vi "InsertQuery.vi"(8 "Error In":errorcluster, 10 "input cluster":T1, 11 "connection reference":T2) -> (0 "Error Out":errorcluster, 2 "Result_2D":string[][](array[string]), 4 "Result_1D":string[](array[string]), 5 "Element":string, 6 "Result_1D Row":string[](array[string]))   [LabVIEW 2020]
uses:
  <vilib>/addons/database/Connection.llb/Conn ObjectReference.ctl
  crearQry.dll
  <vilib>/addons/database/Connection.llb/Conn Execute.vi
  <vilib>/addons/database/Recordset.llb/Rec Fetch Recordset Data (R).vi
  <vilib>/addons/database/Recordset.llb/Rec Destroy - Connection.vi
  <vilib>/addons/database/_DB Variant To Data/Database Variant To Data.xnode
  <vilib>/addons/database/NI_Database_API.lvlib
panel:
  out "Records":i32
  out "sqlQry":string
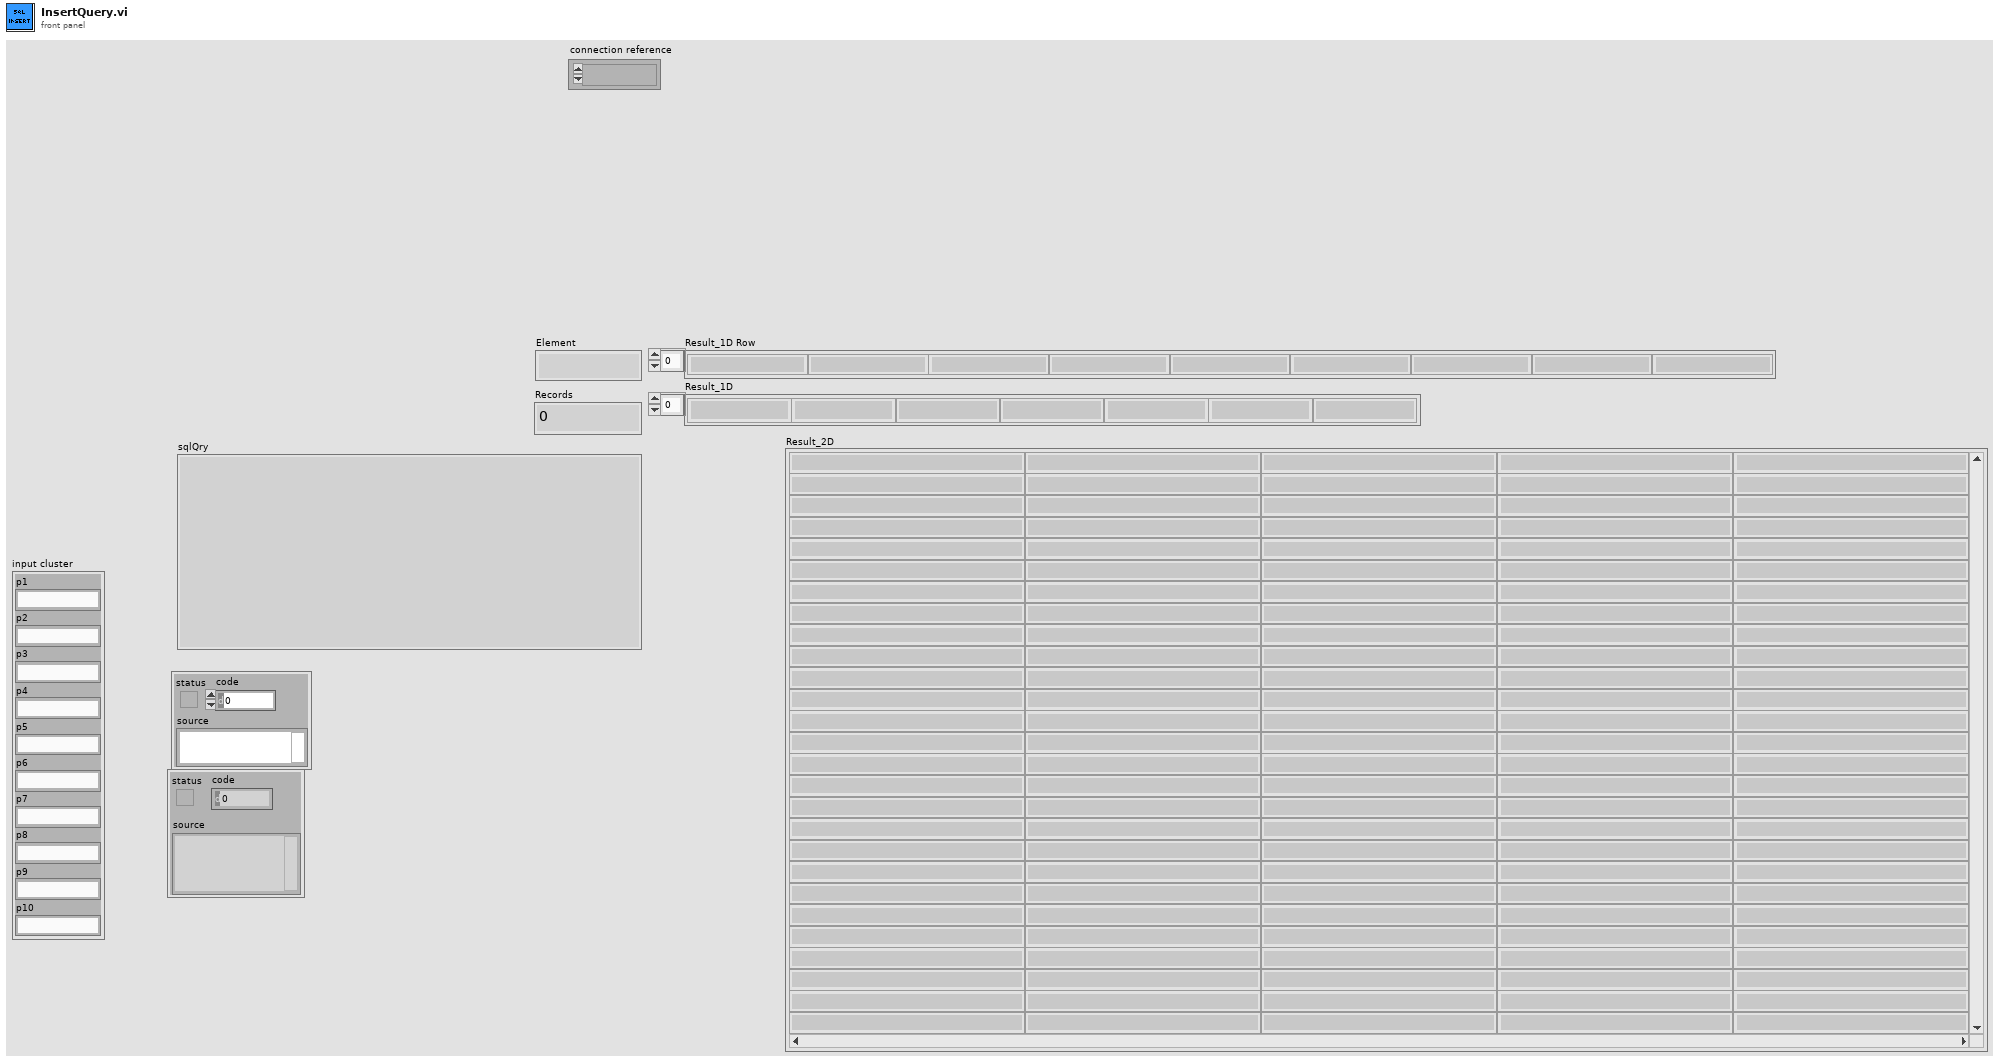
[diagram p1: front panel]
types:
  T1 = cluster{"p1":string, "p2":string, "p3":string, "p4":string, "p5":string, "p6":string, "p7":string, "p8":string, "p9":string, "p10":string}
  T2 = typedef "NI_Database_API.lvlib/Conn ObjectReference.ctl" = refnum<k1>
  T3 = typedef "NI_Database_API.lvlib/Rec ObjectReference.ctl" = refnum<k1>
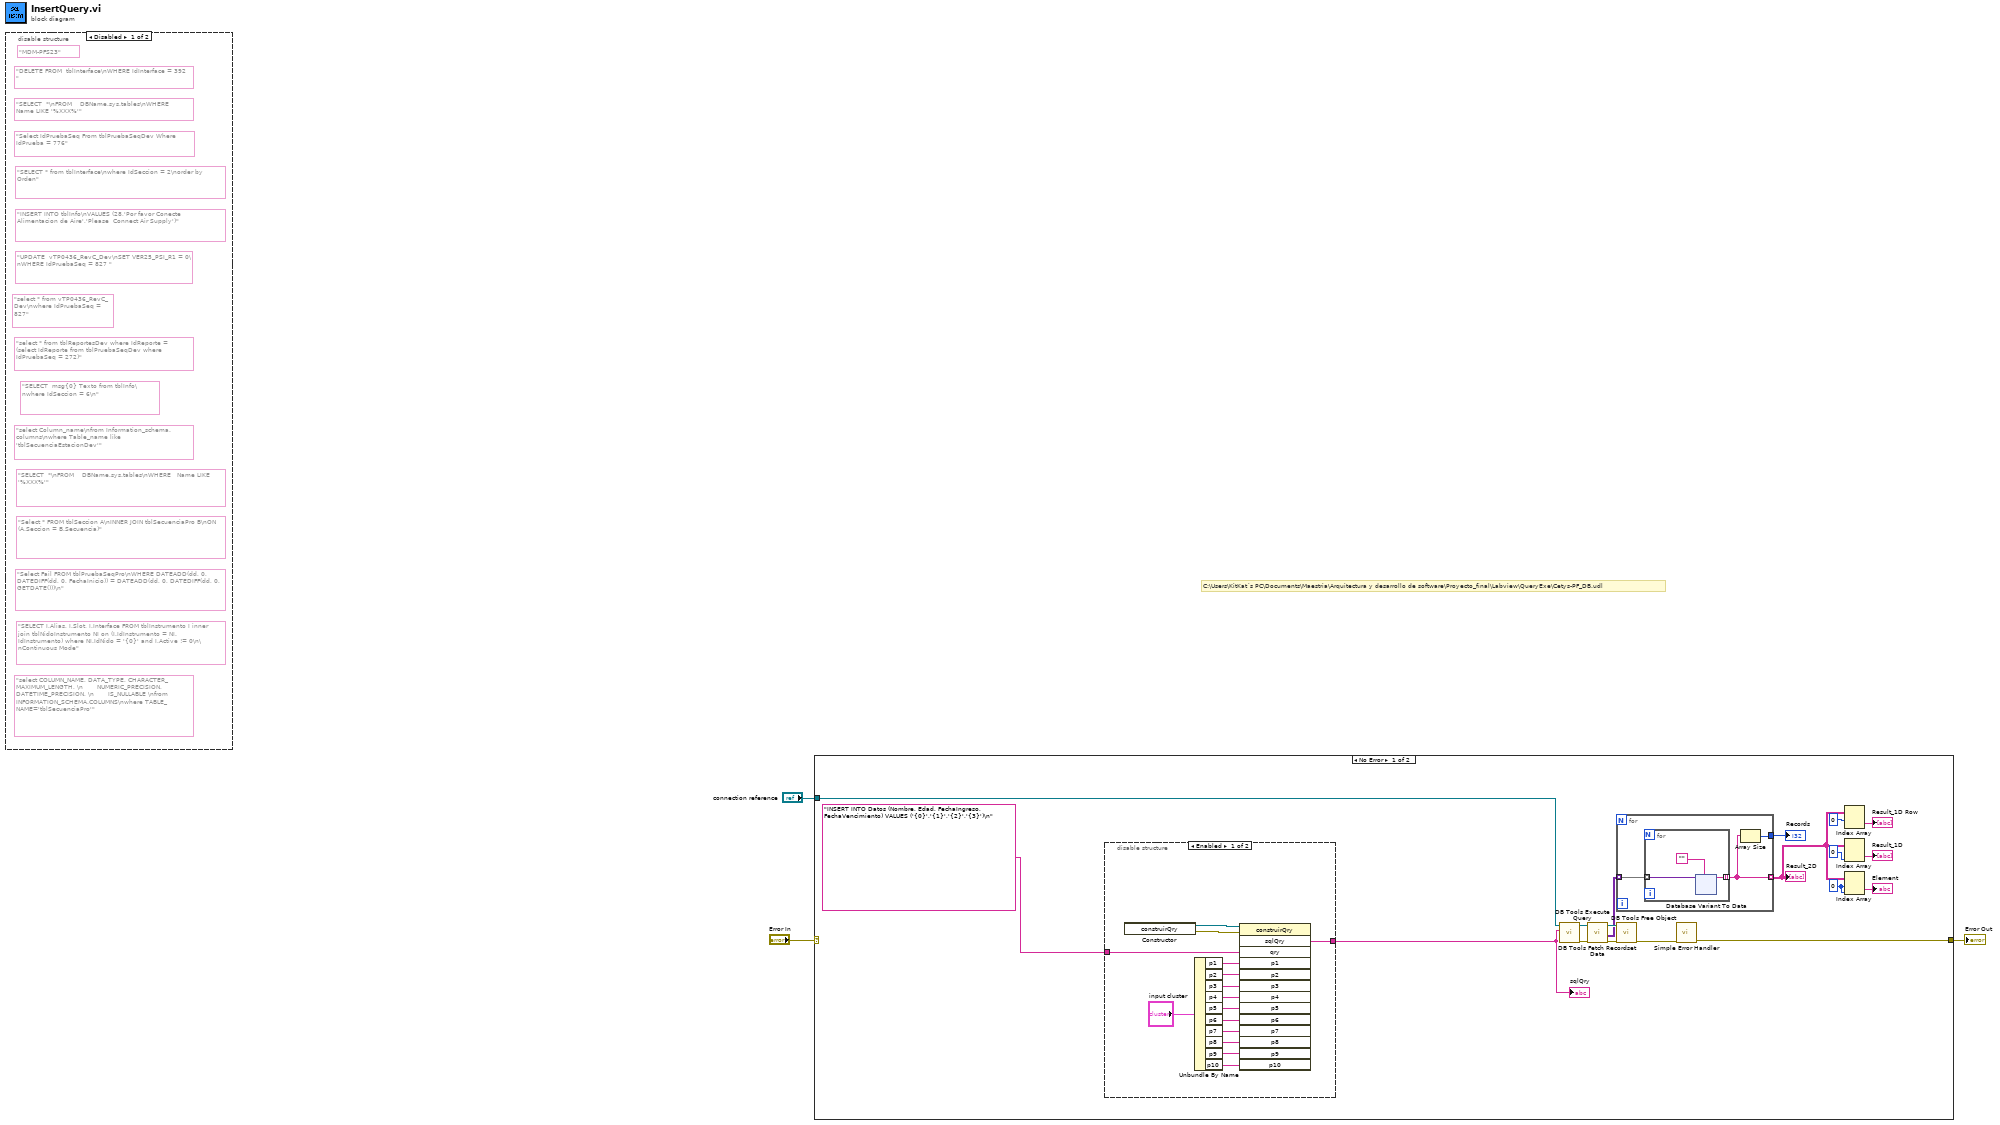
[diagram p0: block diagram]
diagram:
  # "C:\\Users\\KitKat´s PC\\Documents\\Maestria\\Arquitectura y desarrollo de software\\Proyecto_final\\Labview\\QueryExe\\Cetys-PF_DB.udl"
  n1 = disable-structure shown="Disabled" {
    frame Disabled {
      (unwired) "SELECT  msg{0} Texto from tblInfo\nwhere IdSeccion = 6\n" ("qry")
      (unwired) "select * from vTP0436_RevC_Dev\nwhere IdPruebaSeq = 827" ("qry")
      (unwired) "MDM-PFS23" ("Nombre de PC")
      (unwired) "SELECT  *\nFROM    DBName.sys.tables\nWHERE   Name LIKE '%XXX%'" ("qry")
      (unwired) "Select Fail FROM tblPruebaSeqPro\nWHERE DATEADD(dd, 0, DATEDIFF(dd, 0, FechaInicio)) = DATEADD(dd, 0, DATEDIFF(dd, 0, GETDATE()))\n" ("qry")
      (unwired) "Select * FROM tblSeccion A\nINNER JOIN tblSecuenciaPro B\nON (A.Seccion = B.Secuencia)" ("qry")
      (unwired) "SELECT * from tblInterface\nwhere IdSeccion = 2\norder by Orden" ("qry")
      (unwired) "SELECT I.Alias, I.Slot, I.Interface FROM tblInstrumento I inner join tblNidoInstrumento NI on (I.IdInstrumento = NI.IdInstrumento) where NI.IdNido = '{0}' and I.Active != 0\n\nContinuous Mode" ("qry")
      (unwired) "select * from tblReportesDev where IdReporte = (select IdReporte from tblPruebaSeqDev where IdPruebaSeq = 272)" ("sqlQry")
      (unwired) "DELETE FROM  tblInterface\nWHERE IdInterface = 392 " ("qry")
      (unwired) "select COLUMN_NAME, DATA_TYPE, CHARACTER_MAXIMUM_LENGTH, \n       NUMERIC_PRECISION, DATETIME_PRECISION, \n       IS_NULLABLE \nfrom INFORMATION_SCHEMA.COLUMNS\nwhere TABLE_NAME='tblSecuenciaPro'" ("qry")
      (unwired) "SELECT  *\nFROM    DBName.sys.tables\nWHERE   Name LIKE '%XXX%'" ("qry")
      (unwired) "select Column_name\nfrom Information_schema.columns\nwhere Table_name like 'tblSecuenciaEstacionDev'" ("qry")
      (unwired) "Select IdPruebaSeq From tblPruebaSeqDev Where IdPrueba = 776" ("qry")
      (unwired) "UPDATE  vTP0436_RevC_Dev\nSET VER25_PSI_R1 = 0\nWHERE IdPruebaSeq = 827 " ("qry")
      (unwired) "INSERT INTO tblInfo\nVALUES (28,'Por favor Conecte Alimentacion de Aire','Please  Connect Air Supply')" ("qry")
    }
    frame Enabled {
    }
  }
  n2 = case shown="No Error" "Error In" {
    selector: "Error In" -> [_ w75]
    tunnel: [w17 w75] -> w3
    tunnel: "connection reference" -> [w7 _]
    frame No Error {
      w14 = 0 ("index (row)")
      n3 = disable-structure shown="Enabled" {
        disable-tunnel: [w34 _] -> w5
        disable-tunnel: "INSERT INTO Datos (Nombre, Edad, FechaIngreso, FechaVencimiento) VALUES ('{0}','{1}','{2}','{3}')\n" ("qry") -> [w23 _]
        frame Enabled {
          n4 = constructor class="construirQry"() -> (reference out=w36:refnum<k24>, error out=w35:errorcluster)  [unwired: 3 in, 1 out]
          n5 = Unbundle By Name("input cluster") -> ("p1"=w33:string, "p2"=w32:string, "p3"=w31:string, "p4"=w30:string, "p5"=w29:string, "p6"=w28:string, "p7"=w27:string, "p8"=w26:string, "p9"=w25:string, "p10"=w24:string)
          n6 = invoke class="construirQry" method="sqlQry"(reference=w36, error in=w35, "qry"=w23, "p1"=w33, "p2"=w32, "p3"=w31, "p4"=w30, "p5"=w29, "p6"=w28, "p7"=w27, "p8"=w26, "p9"=w25, "p10"=w24) -> ("sqlQry"=w34:string)  [unwired: 1 in, 13 out]
        }
        frame Disabled {
        }
      }
      "sqlQry" <- w5
      n7 = call-poly <vilib>:"DB Tools Execute Query.vi"("SQL query"=w5, "connection reference"=w7) -> ("error out"=w20:errorcluster, "recordset reference"=w21:T3)  [unwired: 6 in]
      n8 = call-poly <vilib>:"DB Tools Fetch Recordset Data.vi"("error in (no error)"=w20, "recordset reference"=w21) -> ("error out"=w18:errorcluster, "recordset data"=w16:variant[][], "recordset reference out"=w19:T3)  [unwired: 3 in]
      n9 = for {
        tunnel: w16 -> [w39] mode=indexing
        tunnel: [w38] -> w10 mode=indexing
        tunnel: [w37] -> w15
        n10 = for {
          tunnel: w39 -> [w42] mode=indexing
          tunnel: [w41] -> w38 mode=indexing
          n11 = xnode "Database Variant To Data"("database variant"=w42, "type"="") -> ("data"=w41:string)  [unwired: 1 in, 1 out]
        }
        n12 = Array Size(array=w38) -> (size(s)=w37:i32)
      }
      "Result_2D" <- w10
      "Records" <- w15
      n13 = call-poly <vilib>:"DB Tools Free Object.vi"("error in (no error)"=w18, "recordset reference"=w19) -> ("error out"=w6:errorcluster)  [unwired: 8 in, 1 out]
      n14 = call <vilib>:"Simple Error Handler.vi"("error in (no error)"=w6) -> ("error out"=w17:errorcluster)  [unwired: 4 in, 4 out]
      n15 = Index Array(array=w10, index (row)=0 ("disabled index (col)")) -> (element=→"Result_1D Row":string[])  [unwired: 1 in]
      n16 = Index Array(array=w10, index (col)=0 ("disabled index (col)")) -> (element=→"Result_1D":string[])  [unwired: 1 in]
      n17 = Index Array(array=w10, index (row)=w14, index (col)=w14) -> (element=→"Element":string)
    }
    frame Error {
    }
  }
  "Error Out" <- w3
